vi "U6 easy Stream Full with loop time analysis.vi"() -> ()   [LabVIEW 2021]
panel:
  out "Processing Time [ms]":i32=1
  out "Graph Update Time [ms]":i32=1
  out "Stream Read Time [ms]":i32=1
  out "Loop Time [ms]":i32=1
  in  "Simulated Processing Delay [ms]":u32
  in  "Iterations/Second":i32=1
  in  "Binary":bool
  in  "StreamSettlingFactor":i32
  in  "Resolution Index":u8
  in  "Range Constants":u8[](array[ring])=[0, 0, 0, 0] items=["LJ_rgBIP10V", "LJ_rgBIP1V", "LJ_rgBIPP1V", "LJ_rgBIPP01V"]
  out "Stream Parameters":T1 {"Device Backlog [%]" format="%.2f"}
  in  "PC buffer size (seconds)":dbl=10.0 format="%.2f"
  in  "Scan List (-)":u8[](array[numeric])=[199, 199, 199, 199]
  out "Data":dbl[][](array[numeric]) format="%.3f"
  out "Waveform Graph":dbl[][](graph)
  in  "Scan List (+)":u8[](array[numeric])=[0, 1, 2, 3]
  out "# of iterations":i32
  in  "Scan Rate (Hz)":dbl=1000.0 format="%.3f"
  in  "stop":bool
  out "Error Message":string
  # "This example streams from the first found USB U6."
  # "The + scan list is the positive\nchannels.  For each element in\nthe + list, there must also be\nan element in the - list, which is\nthe negative channels.  For\nsingle-ended channels, put in\n199 for the negative channel.\n\nTo remove an element, right-click\non it, select Data Operations =>\nRemove Element.\n\nTo empty an array, right-click\nnear the edge, select Data\nOperations => Empty Array.\n\nOther useful operations:  From the\nOperate menu are \"Make Current\nValues Default\" and \"Reinitialize\nTo Default\"."
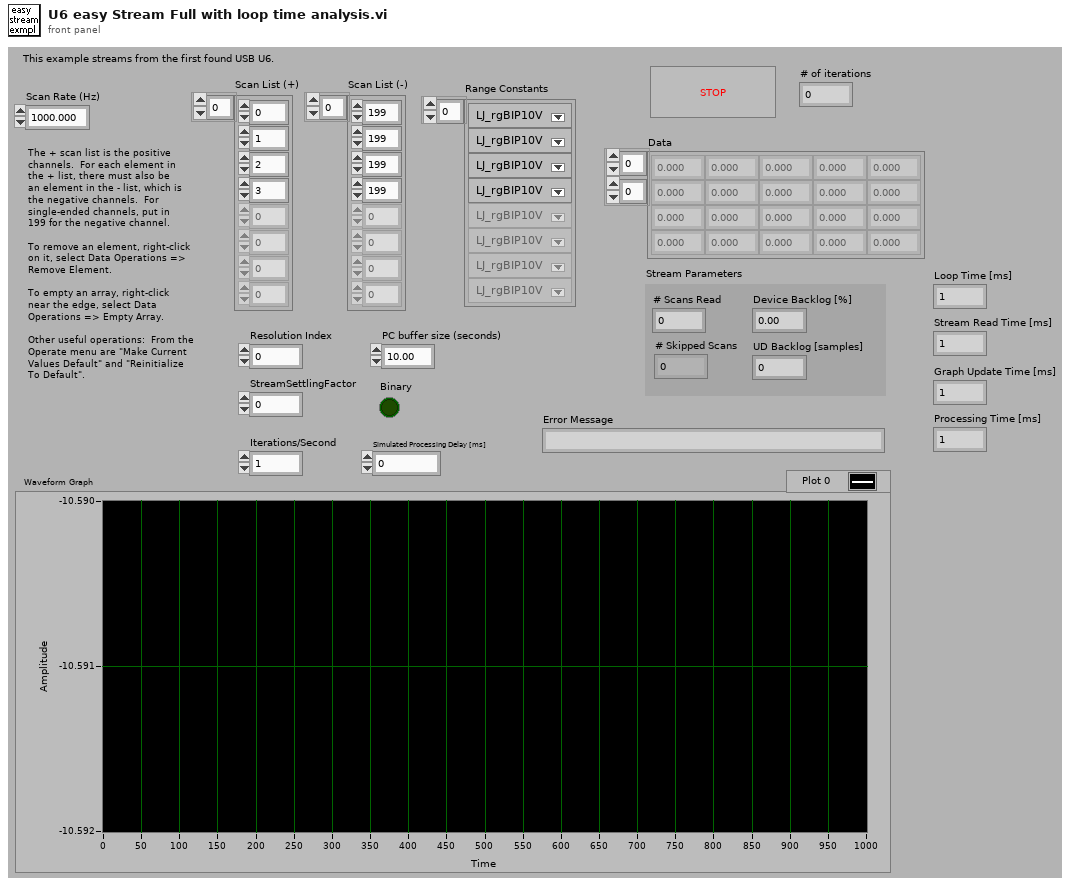
[diagram p1: front panel]
types:
  T1 = cluster{"# Scans Read":i32, "# Skipped Scans":i32, "Device Backlog [%]":dbl, "UD Backlog [samples]":i32}
  T2 = cluster{"PC buffer size (seconds)":dbl, "Resolution Index":u8, "StreamSettlingFactor":i32, "Binary":bool}
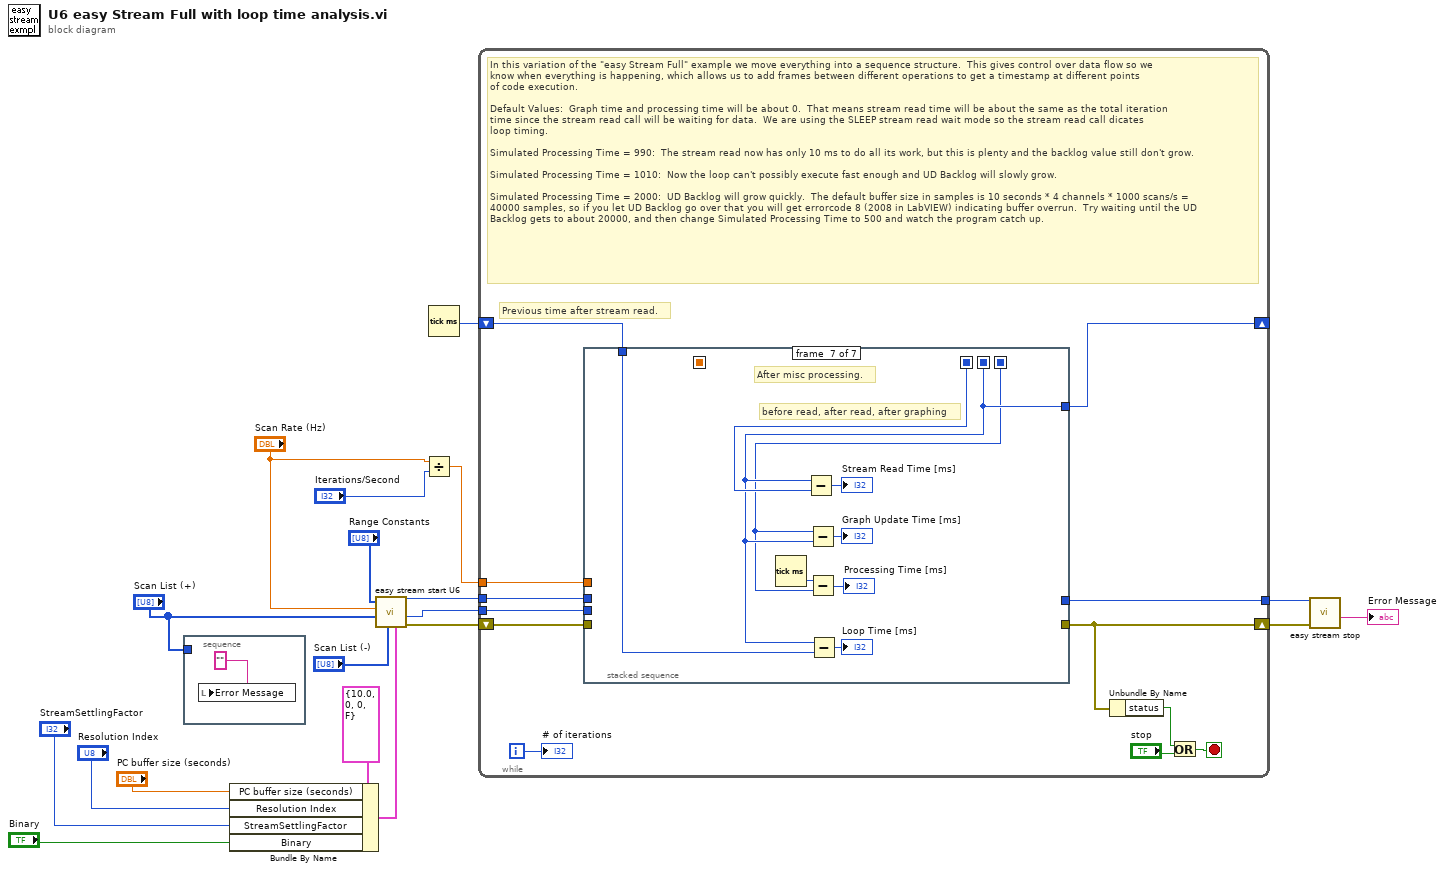
[diagram p0: block diagram]
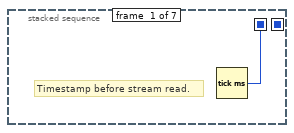
[diagram p2: hidden frame]
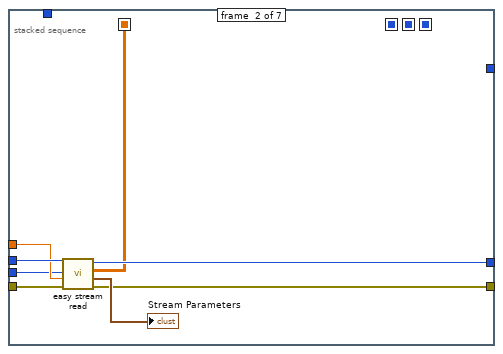
[diagram p3: hidden frame]
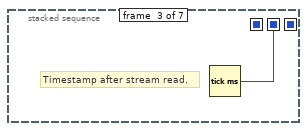
[diagram p4: hidden frame]
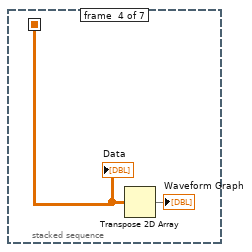
[diagram p5: hidden frame]
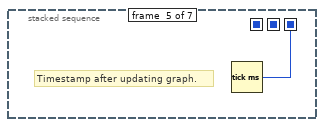
[diagram p6: hidden frame]
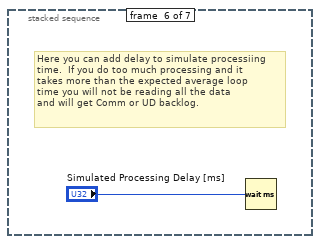
[diagram p7: hidden frame]
diagram:
  n1 = stacked-sequence {
    tunnel: "Scan List (+)" -> [_]
    frame #0 {
      n2 = local write "Error Message"("" ("Error Message")) -> ()
    }
  }
  n3 = Bundle By Name(cluster=T2 {"PC buffer size (seconds)"=10.0, "Resolution Index"=0, "StreamSettlingFactor"=0, "Binary"=FALSE} ("Advanced"), "PC buffer size (seconds)"="PC buffer size (seconds)", "Resolution Index"="Resolution Index", "StreamSettlingFactor"="StreamSettlingFactor", "Binary"="Binary") -> (w9:T2)
  n4 = call "easy stream start U6.vi"("Advanced"=w9, "Scan List (-)"="Scan List (-)", "Scan List (+)"="Scan List (+)", "Scan Rate (Hz)"="Scan Rate (Hz)", "Range Constants"="Range Constants") -> ("error out"=w19:errorcluster, "# Channels"=w18:i32, "Handle Out"=w17:i32)  [unwired: 3 in, 1 out]
  n5 = Divide(x="Scan Rate (Hz)", y="Iterations/Second") -> (x/y=w2:dbl)
  n6 = Tick Count (ms)() -> (millisecond timer value=w1:u32)
  n7 = while {
    tunnel: [w28] -> w15
    tunnel: w17 -> [w26]
    tunnel: w18 -> [w21]
    shift-left: w19 -> [w27]
    shift-right: [w22] -> w16
    tunnel: w2 -> [w25]
    shift-right: [w24] -> _
    shift-left: w1 -> [w23]
    i -> [w29]
    stop <- w30 stop-if-true
    # "In this variation of the \"easy Stream Full\" example we move everything into a sequence structure.  This gives control over data flow so we\nknow when everything is happening, which allows us to add frames between different operations to get a timestamp at different points\nof code execution.\n\nDefault Values:  Graph time and processing time will be about 0.  That means stream read time will be about the same as the total iteration\ntime since the stream read call will be waiting for data.  We are using the SLEEP stream read wait mode so the stream read call dicates\nloop timing.\n\nSimulated Processing Time = 990:  The stream read now has only 10 ms to do all its work, but this is plenty and the backlog value still don't grow.\n\nSimulated Processing Time = 1010:  Now the loop can't possibly execute fast enough and UD Backlog will slowly grow.\n\nSimulated Processing Time = 2000:  UD Backlog will grow quickly.  The default buffer size in samples is 10 seconds * 4 channels * 1000 scans/s =\n40000 samples, so if you let UD Backlog go over that you will get errorcode 8 (2008 in LabVIEW) indicating buffer overrun.  Try waiting until the UD\nBacklog gets to about 20000, and then change Simulated Processing Time to 500 and watch the program catch up."
    # "Previous time after stream read."
    n8 = stacked-sequence {
      seq-local: [_ w35 _ _ _ _ _] -> [_ _ _ w43 _ _ _]
      seq-local: [w33 _ _ _ _ _ _] -> [_ _ _ _ _ _ w49]
      seq-local: [_ _ w42 _ _ _ _] -> [_ _ _ _ _ _ w48]
      seq-local: [_ _ _ _ w45 _ _] -> [_ _ _ _ _ _ w47]
      tunnel: [_ w39 _ _ _ _ _] -> w22
      tunnel: [_ w37 _ _ _ _ _] -> w28
      tunnel: w27 -> [_ w40 _ _ _ _ _]
      tunnel: w26 -> [_ w38 _ _ _ _ _]
      tunnel: w25 -> [_ w36 _ _ _ _ _]
      tunnel: [_ _ _ _ _ _ w48] -> w24
      tunnel: w23 -> [_ _ _ _ _ _ w51]
      tunnel: w21 -> [_ w34 _ _ _ _ _]
      frame #0 {
        # "Timestamp before stream read."
        n9 = Tick Count (ms)() -> (millisecond timer value=w33:u32)
      }
      frame #1 {
        n10 = call "easy stream read.vi"("error in"=w40, "Scans To Read"=w36, "# Channels In Stream"=w34, "Handle In"=w38) -> ("error out"=w39:errorcluster, "Stream Parameters"=→"Stream Parameters":T1, "Data"=w35:dbl[][], "Handle Out"=w37:i32)  [unwired: 4 in]
      }
      frame #2 {
        # "Timestamp after stream read."
        n11 = Tick Count (ms)() -> (millisecond timer value=w42:u32)
      }
      frame #3 {
        n12 = Transpose 2D Array(2D array=w43) -> (transposed array=→"Waveform Graph":dbl[][])
        "Data" <- w43
      }
      frame #4 {
        # "Timestamp after updating graph."
        n13 = Tick Count (ms)() -> (millisecond timer value=w45:u32)
      }
      frame #5 {
        # "Here you can add delay to simulate processiing\ntime.  If you do too much processing and it\ntakes more than the expected average loop\ntime you will not be reading all the data\nand will get Comm or UD backlog."
        n14 = Wait (ms)(milliseconds to wait="Simulated Processing Delay [ms]") -> ()  [unwired: 1 out]
      }
      frame #6 {
        # "After misc processing."
        # "before read, after read, after graphing"
        n15 = Tick Count (ms)() -> (millisecond timer value=w50:u32)
        n16 = Subtract(x=w48, y=w49) -> (x-y=→"Stream Read Time [ms]":u32)
        n17 = Subtract(x=w47, y=w48) -> (x-y=→"Graph Update Time [ms]":u32)
        n18 = Subtract(x=w50, y=w47) -> (x-y=→"Processing Time [ms]":u32)
        n19 = Subtract(x=w48, y=w51) -> (x-y=→"Loop Time [ms]":u32)
      }
    }
    n20 = Unbundle By Name(w22) -> ("status"=w31:bool)
    n21 = Or(x=w31, y="stop") -> (x .or. y?=w30:bool)
    "# of iterations" <- w29
  }
  n22 = call "easy stream stop.vi"("error in"=w16, "Handle In"=w15) -> ("Error Message"=→"Error Message":string)  [unwired: 7 in, 2 out]
